vi "1D Polynomial Evaluation (DBL).vi"(2 "P(x)":dbl[](array[numeric]) min=0.0 max=127.0 format="%#.2f", 3 "A":dbl[](array[numeric])) -> (0 "error":i32, 1 "P(A)":dbl[](array[numeric]))   [LabVIEW 2020, in "NI_AALPro.lvlib"]
doc: "Evaluates the polynomial <B>P(x)</B> with a single value or multiple values. The data types you wire to the <B>a</B> and <B>P(x)</B> inputs determine the polymorphic instance to use."
uses:
  <vilib>/Analysis/NI_AALPro.lvlib
  <vilib>/Analysis/polynomials.llb/Remove Zero Coefficients (DBL).vi
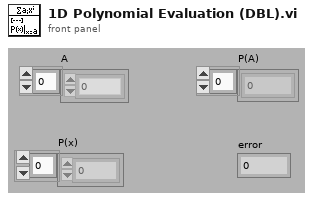
[diagram p1: front panel]
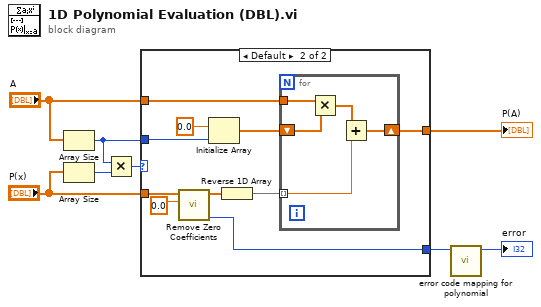
[diagram p0: block diagram]
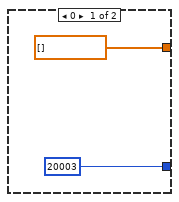
[diagram p2: hidden frame]
diagram:
  n1 = Array Size(array="A") -> (size(s)=w3:i32)
  n2 = Array Size(array="P(x)") -> (size(s)=w6:i32)
  n3 = Multiply(x=w3, y=w6) -> (x*y=w5:i32)
  n4 = case shown="Default" w5 {
    tunnel: "P(x)" -> [_ w16]
    tunnel: "A" -> [_ w19]
    tunnel: [dbl[] [] w18] -> w8
    tunnel: [20003 ("empty array") w14] -> w2
    tunnel: w3 -> [_ w12]
    frame 0 {
    }
    frame Default {
      n5 = call-poly <vilib>:"Remove Zero Coefficients.vi"("threshold"=0.0, "P(x) In"=w16) -> ("error"=w14:i32, "P(x) Out"=w15:dbl[])  [unwired: 7 in, 1 out]
      n6 = Initialize Array(0.0, w12) -> (w11:dbl[])
      n7 = Reverse 1D Array(array=w15) -> (reversed array=w20:dbl[])
      n8 = for {
        shift-right: [w21] -> w18
        shift-left: w11 -> [w24]
        tunnel: w19 -> [w25]
        tunnel: w20 -> [w23] mode=indexing
        n9 = Multiply(x=w25, y=w24) -> (x*y=w22:dbl[])
        n10 = Add(x=w22, y=w23) -> (x+y=w21:dbl[])
      }
    }
  }
  "P(A)" <- w8
  n11 = call <vilib>:"error code mapping for polynomial.vi"("error in"=w2) -> ("error out"=→"error":i32)  [unwired: 10 in]
